vi "Main.vi"() -> ()   [LabVIEW 2021, in "Game of Life.lvlib"]
doc: "This template is for the Queued Message Handler design pattern.\n\nThe Event Handling Loop generates messages based on user interface actions.\n\nThe Message Handling Loop processes messages generated by the Event Handling Loop, or by other messages. The messages are string values, so new messages can be added easily to the Message Cases case structure in the Message Handling Loop. Each message cluster can also provide an optional value for Message Data, which is a variant that can be converted to whatever message-specific data is required."
uses:
  Game of Life.lvlib
  <vilib>/Plug-In SDKs/InstrumentStudio SDK/InstrumentStudioPluginSDK.lvlibp/Plugin Events Enum.ctl
  controls/Data.ctl
  controls/Configuration.ctl
  <vilib>/Utility/error.llb/DialogType.ctl
  controls/Game of Life.ctl
  a2cd5499-92a9-455c-b0f9-1db12e3f6067.vi
  aef85ed4-6d5b-4a62-8cd4-232f16e6ae51.vi
  a2cd5499-92a9-455c-b0f9-1db12e3f6067.vi/6651a77e-856e-4bcd-af5a-c0c13b264cc1.vi
  aef85ed4-6d5b-4a62-8cd4-232f16e6ae51.vi/331b549c-fcf8-43d9-8a1e-5b3c0091a99c.vi
  <vilib>/JDP Science/JSONtext/JSON text to Variant.vi
  <vilib>/Utility/error.llb/Error Cluster From Error Code.vi
  <vilib>/JDP Science/JSONtext/Variant to JSON Text.vi
  <vilib>/JDP Science/JSONtext/LVClass Serializer/JSONtext LVClass Serializer.lvclass
  <vilib>/ErrorRing/Error Ring.xnode
  <vilib>/Plug-In SDKs/InstrumentStudio SDK/InstrumentStudioPluginSDK.lvlibp/Plugin Session.lvclass
  <vilib>/Plug-In SDKs/InstrumentStudio SDK/InstrumentStudioPluginSDK.lvlibp
panel:
  in  "Tab Control":enum32{"Game Panel", "Events"}(tab)
  in  "Start/Stop":bool
  out "game of life":T1(graph)
  out "generation":u32 caption="Generation"
  in  "update interval":u32=250 caption="Update interval (msec)" min=50 max=1000
  in  "height":u32=100 caption="Board height" min=10
  in  "width":u32=100 caption="Board width" min=10
  in  "Log Events?":bool caption="Enable Logging"
  out "Event Record":i32(listbox)
  out "Log file directory":path
  in  "Session Id":u64
  # "When logging is enabled, a log file will be generated in the specified \ndirectory after the front panel is closed."
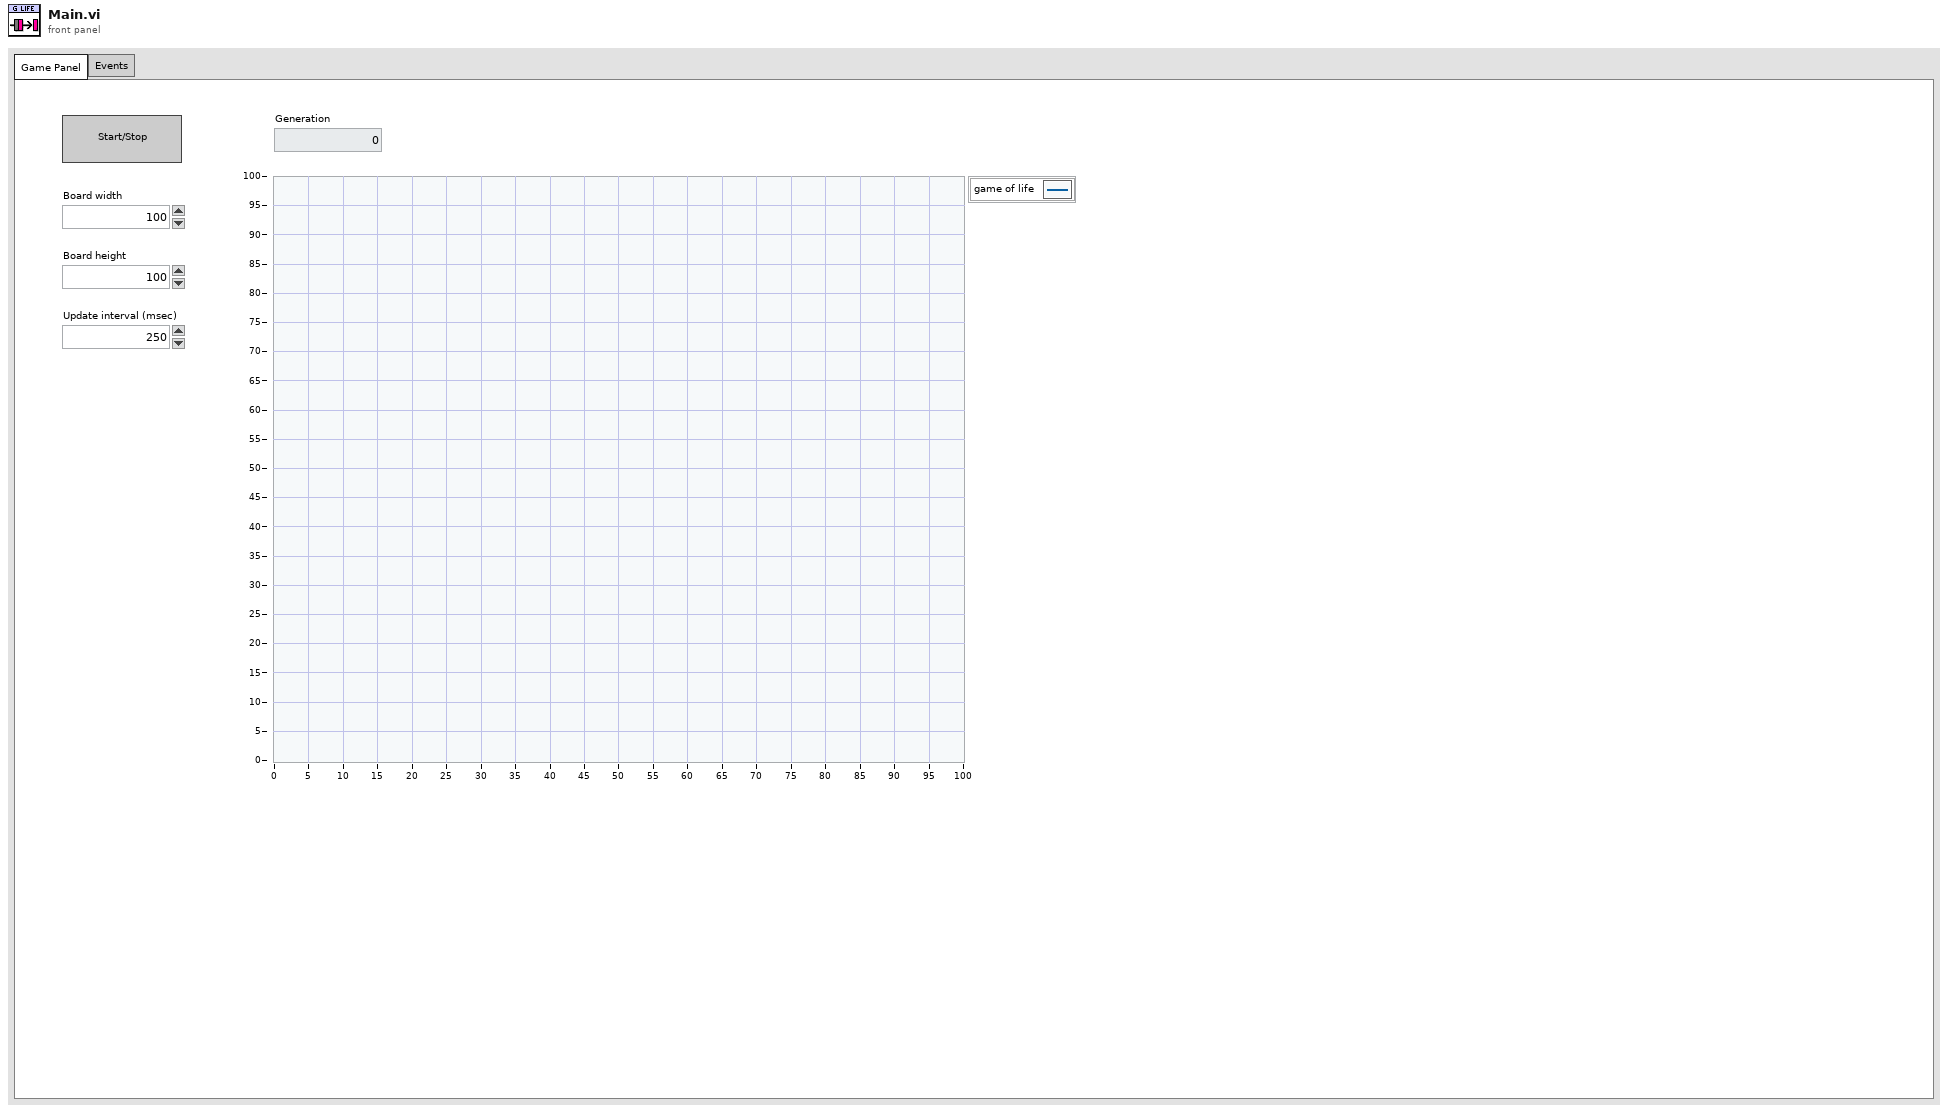
[diagram p1: front panel]
types:
  T1 = typedef "Game of Life.lvlib/Game of Life.ctl" = cluster{"x_data":dbl[], "y_data":dbl[]}
  T2 = typedef "Game of Life.lvlib/Data.ctl" = cluster{"Configuration":T3, "Generation":u32, "Item Names":string[], "Run?":bool, "Cells":bool[][]}
  T3 = typedef "Game of Life.lvlib/Configuration.ctl" = cluster{"Height":u32, "Width":u32, "Interval":u32, "Log Path":path, "Log Events?":bool}
  T4 = typedef "InstrumentStudioPluginSDK.lvlibp/Plugin Events Enum.ctl" = enum16{"Shutdown", "Project Saved", "Stop All Outputs"}
  T5 = typedef "InstrumentStudioPluginSDK.lvlibp/Event Registration Refnum.ctl" = refnum<event-registration>
  T6 = typedef "Game of Life.lvlib/All Message Queues.ctl" = cluster{"UI":refnum<queue>}
  T7 = cluster{"Event Refnum":T5, "Event Registration Refnum":refnum<event-registration>}
  T8 = enum8{"Enabled", "Disabled", "Disabled and Grayed Out"}
  T9 = typedef "DialogType.ctl" = u16
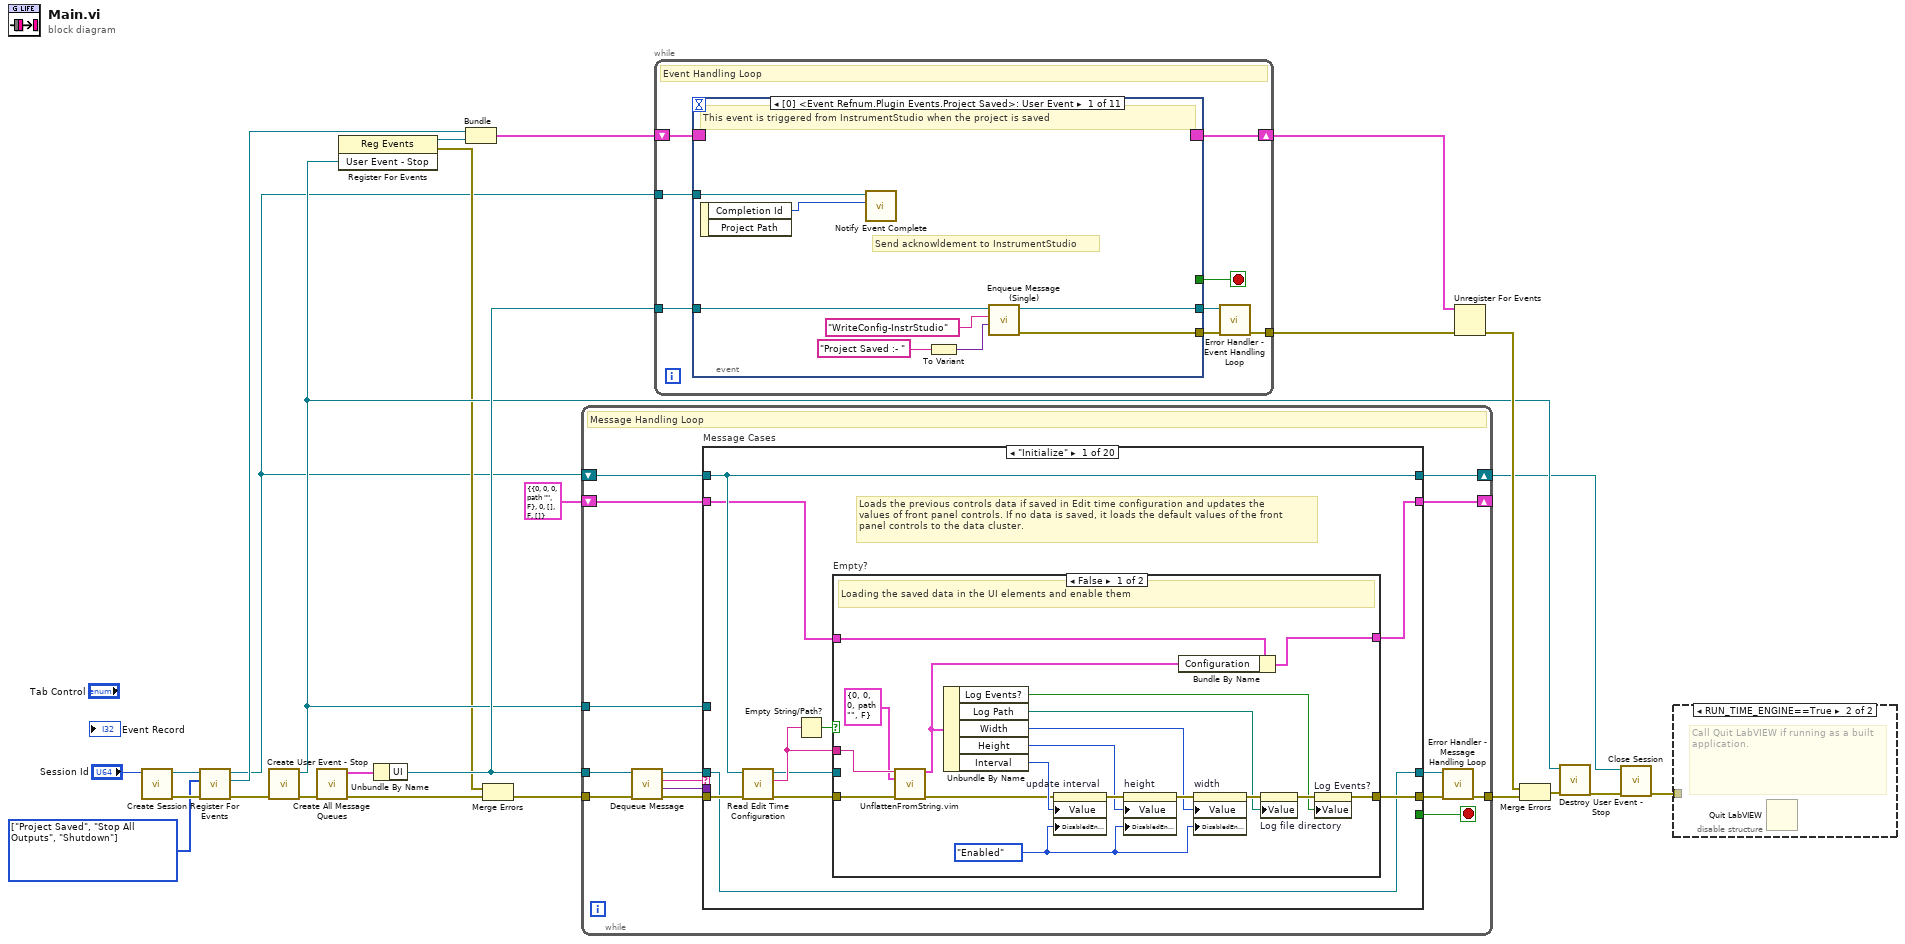
[diagram p0: block diagram]
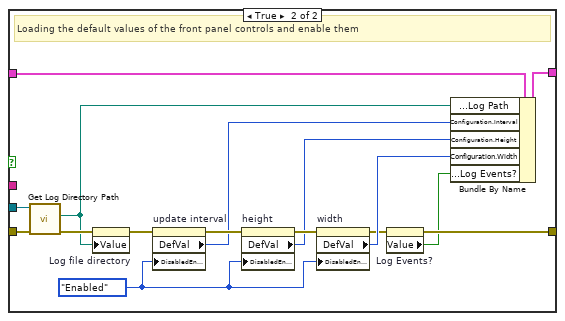
[diagram p3: hidden frame]
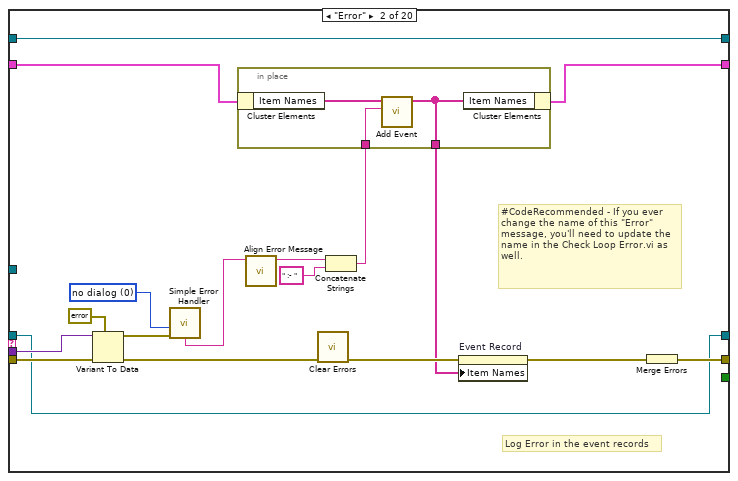
[diagram p4: hidden frame]
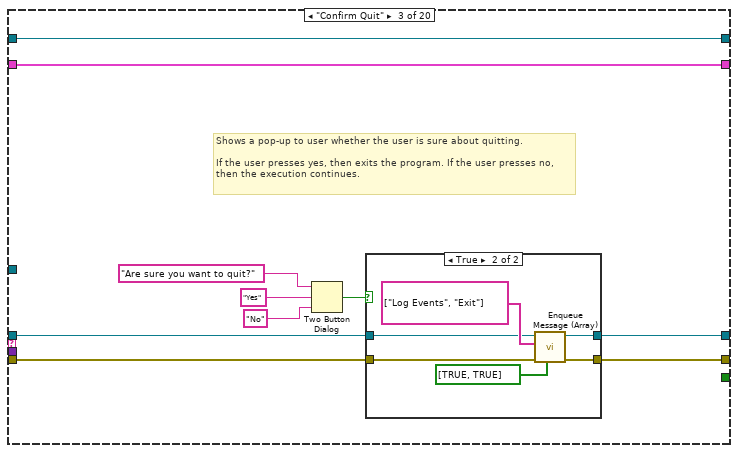
[diagram p5: hidden frame]
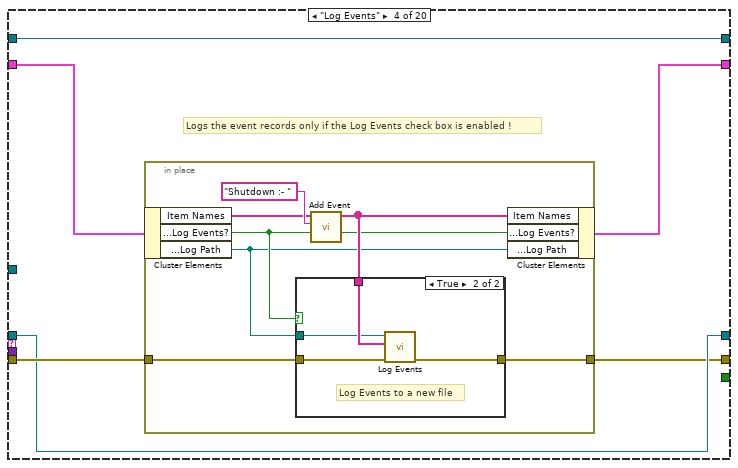
[diagram p7: hidden frame]
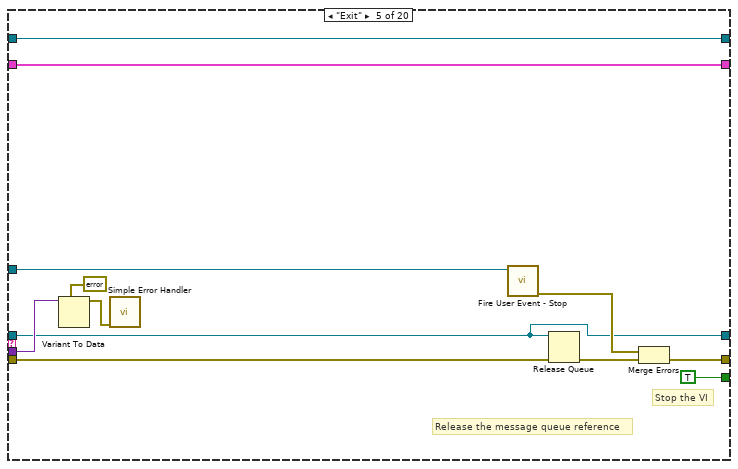
[diagram p9: hidden frame]
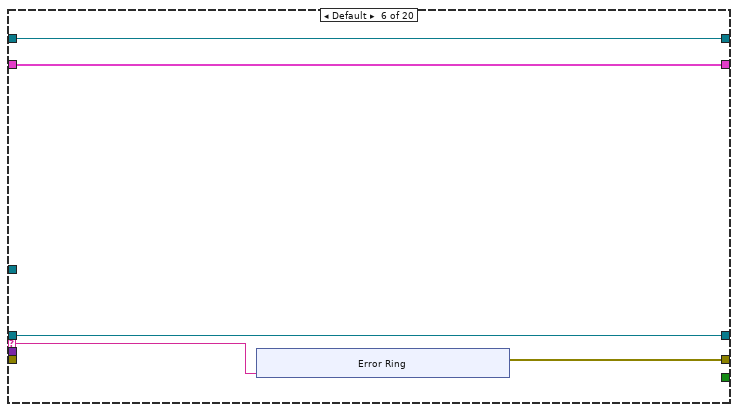
[diagram p10: hidden frame]
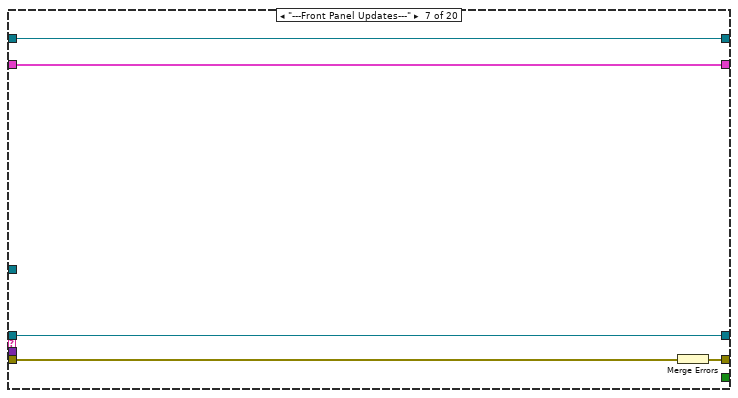
[diagram p11: hidden frame]
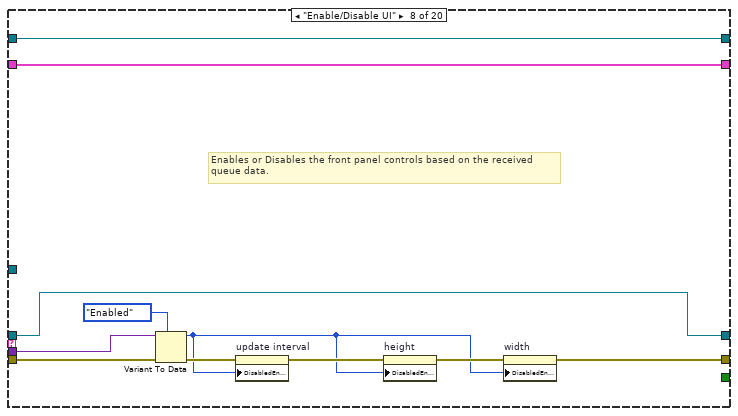
[diagram p12: hidden frame]
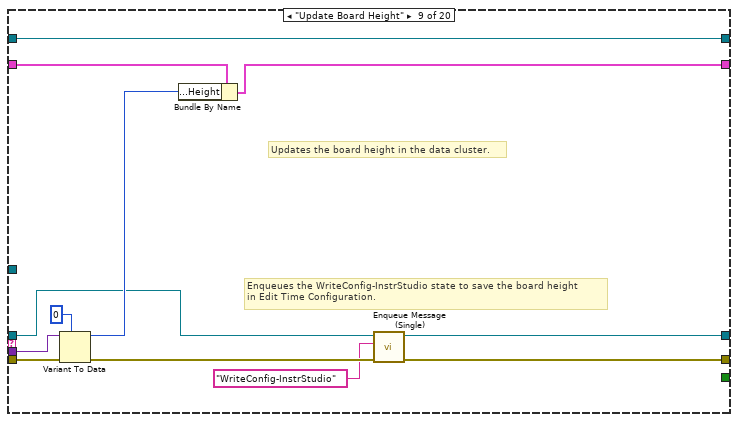
[diagram p13: hidden frame]
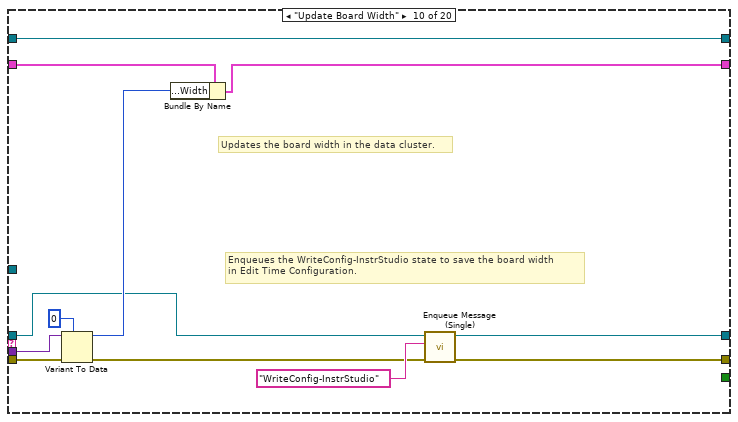
[diagram p14: hidden frame]
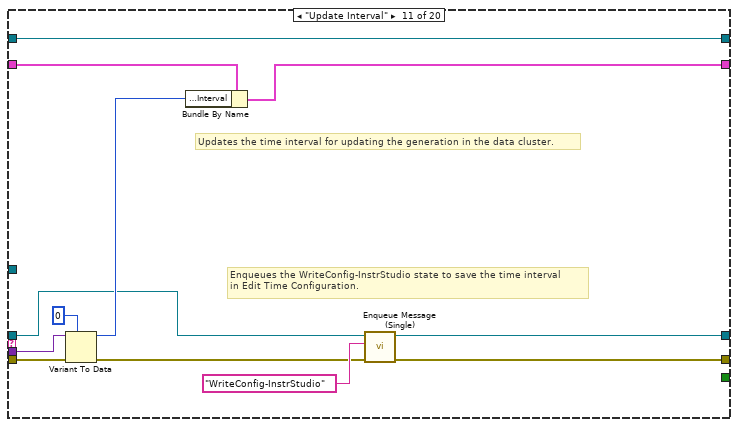
[diagram p15: hidden frame]
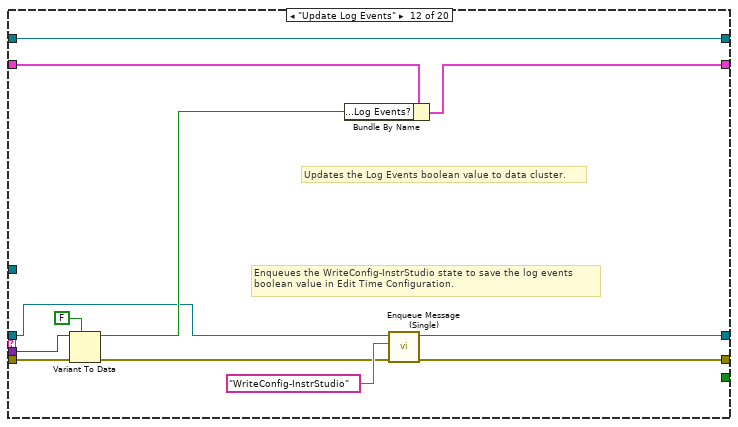
[diagram p16: hidden frame]
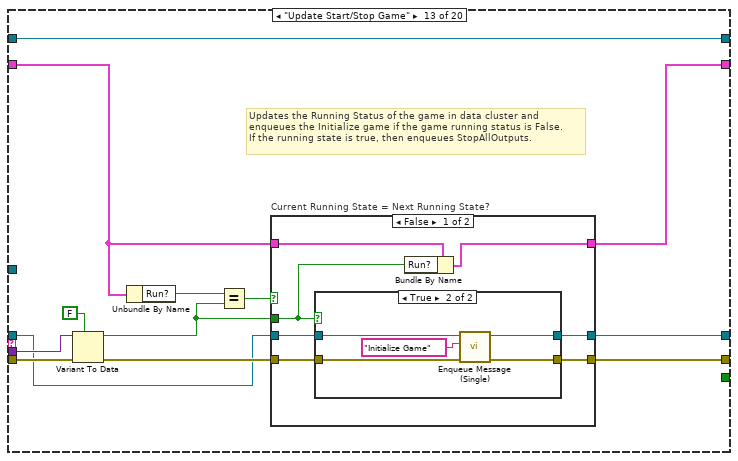
[diagram p17: hidden frame]
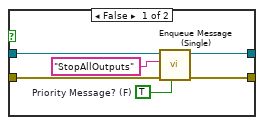
[diagram p18: hidden frame]
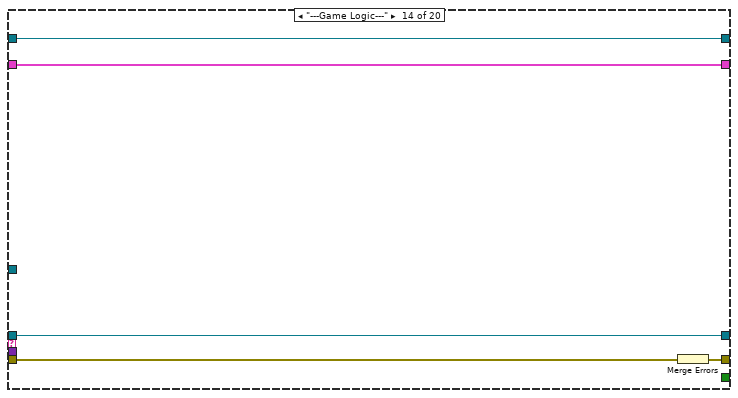
[diagram p20: hidden frame]
diagram:
  w9 = T4[] [enum."Project Saved", enum."Stop All Outputs", enum."Shutdown"] items=["Shutdown", "Project Saved", "Stop All Outputs"] ("Events To Register")
  n1 = call <vilib>:"Create Session.vi"("Session Id"="Session Id") -> ("error out"=w12:errorcluster, "Session out"=w10:refnum<class "Plugin Session.lvclass">)  [unwired: 6 in, 3 out]
  n2 = call <vilib>:"Register For Events.vi"("error in (no error)"=w12, "Events To Register"=w9, "Session in"=w10) -> ("error out"=w11:errorcluster, "Event Refnum"=w6:T5, "Session out"=w2:refnum<class "Plugin Session.lvclass">)  [unwired: 6 in]
  n3 = call "Create User Event - Stop.vi"("error in (no error)"=w11) -> ("error out"=w21:errorcluster, "User Event - Stop"=w16:refnum<user-event>)  [unwired: 9 in]
  n4 = call "Create All Message Queues.vi"("error in (no error)"=w21) -> ("error out"=w25:errorcluster, "Message Queues out"=w24:T6)  [unwired: 9 in]
  n5 = register-events(w16) -> (reference out=w8:refnum<event-registration>, error out=w14:errorcluster)  [unwired: 2 in]
  n6 = Unbundle By Name(w24) -> ("UI"=w22:refnum<queue>)
  n7 = Bundle("Event Refnum"=w6, "Event Registration Refnum"=w8) -> (w7:T7)  [unwired: 1 in]
  n8 = Merge Errors(w14, w25) -> (w15:errorcluster)
  n9 = while {
    tunnel: w22 -> [w34]
    tunnel: w16 -> [w39]
    tunnel: w15 -> [w38]
    tunnel: [w32] -> w23
    shift-right: [w29] -> w5
    shift-left: w2 -> [w30]
    shift-right: [w28] -> _
    shift-left: T2 {"Configuration"={"Height"=0, "Width"=0, "Interval"=0, "Log Path"=path "", "Log Events?"=FALSE}, "Generation"=0, "Item Names"=[], "Run?"=FALSE, "Cells"=[]} ("Configuration") -> [w27]
    stop <- w40 stop-if-true
    # "Message Handling Loop"
    n10 = call "Dequeue Message.vi"("error in (no error)"=w38, "Message Queue"=w34) -> ("error out"=w37:errorcluster, "Message Data"=w35:variant, "Message"=w36:string, "dup Message Queue"=w33:refnum<queue>)  [unwired: 6 in]
    n11 = case "Message Cases" shown="\"Initialize\"" w36 {
      selector: w36 -> [_ _ _ _ _ w157 _ _ _ _ _ _ _ _ _ _ _ _ _ _]
      tunnel: w33 -> [w44 w95 w113 w128 w143 w154 w166 w171 w183 w195 w206 w219 w230 w264 w283 w294 w329 w348 w355 w372]
      tunnel: w37 -> [w46 w102 w115 w129 w142 _ w170 w175 w192 w204 w216 w228 w236 w268 w281 w298 w333 w335 w356 w371]
      tunnel: [w50 w97 w114 w124 w151 w158 w169 w177 w185 w194 w208 w220 w239 w267 w269 w295 w332 w346 w357 w376] -> w31
      tunnel: [_ _ _ _ TRUE _ _ _ _ _ _ _ _ _ _ _ _ _ _ _] -> w40
      tunnel: w35 -> [_ w101 _ _ w146 _ _ w174 w191 w203 w215 w227 w235 _ _ _ _ _ _ w361]
      tunnel: w39 -> [_ _ _ _ w150 _ _ _ _ _ _ _ _ _ _ _ _ _ _ _]
      tunnel: w30 -> [w45 w96 w112 w127 w145 w156 w168 w181 w193 w205 w217 w229 w242 w266 w287 w299 w331 w352 w359 w367]
      tunnel: [w45 w96 w112 w127 w145 w156 w168 w181 w193 w205 w217 w229 w242 w266 w287 w299 w331 w352 w358 w377] -> w29
      tunnel: [w43 w92 w111 w126 w144 w155 w167 w180 w188 w201 w213 w225 w240 w265 w286 w288 w330 w350 w354 w366] -> w28
      tunnel: w27 -> [w42 w91 w111 w125 w144 w155 w167 w180 w187 w200 w212 w224 w241 w265 w285 w292 w330 w339 w354 w365]
      tunnel: [w44 w95 w110 w128 w143 w154 w166 w171 w184 w196 w207 w218 w238 w264 w282 w291 w329 w344 w355 w372] -> w26
      frame "Initialize" {
        # "Loads the previous controls data if saved in Edit time configuration and updates the\nvalues of front panel controls. If no data is saved, it loads the default values of the front\npanel controls to the data cluster."
        # "Initialize - All initialization work should take place in this message, since other loops can potentially enqueue messages that execute immediately after this one."
        n12 = call <vilib>:"Read Edit Time Configuration.vi"("error in (no error)"=w46, "Session in"=w45) -> ("error out"=w47:errorcluster, "Edit Time Configuration"=w48:string, "Session out"=w41:refnum<class "Plugin Session.lvclass">)  [unwired: 7 in]
        n13 = Empty String/Path?(string/path=w48) -> (empty?=w49:bool)
        n14 = case "Empty?" shown="False" w49 {
          tunnel: [w52 w70] -> w50
          tunnel: w47 -> [w67 w74]
          tunnel: w48 -> [w68 _]
          tunnel: w42 -> [w60 w84]
          tunnel: [w59 w80] -> w43
          tunnel: w41 -> [_ w72]
          frame False {
            w56 = T8."Enabled" ("Disabled")
            # "Loading the saved data in the UI elements and enable them"
            n15 = call "UnflattenFromString.vim"("Flattened Data"=w68, "Data Type"=T3 {"Height"=0, "Width"=0, "Interval"=0, "Log Path"=path "", "Log Events?"=FALSE} ("Configuration"), "error in"=w67) -> ("Data Out"=w58:T3, "error out"=w57:errorcluster)  [unwired: 11 in]
            n16 = Unbundle By Name(w58) -> ("Log Events?"=w51:bool, "Log Path"=w54:path, "Width"=w62:u32, "Height"=w64:u32, "Interval"=w66:u32)
            n17 = property on="update interval" class="DigNum (strict)"(error in=w57, "Value"=w66, "DisabledEnum"=w56) -> (error out=w65:errorcluster)  [unwired: 1 in, 1 out]
            n18 = property on="height" class="DigNum (strict)"(error in=w65, "Value"=w64, "DisabledEnum"=w56) -> (error out=w63:errorcluster)  [unwired: 1 in, 1 out]
            n19 = Bundle By Name(cluster=w60, "Configuration"=w58) -> (w59:T2)
            n20 = property on="width" class="DigNum (strict)"(error in=w63, "Value"=w62, "DisabledEnum"=w56) -> (error out=w55:errorcluster)  [unwired: 1 in, 1 out]
            n21 = property on="Log file directory" class="Path"(error in=w55, "Value"=w54) -> (error out=w53:errorcluster)  [unwired: 1 in, 1 out]
            n22 = property on="Log Events?" class="Bool (strict)"(error in=w53, "Value"=w51) -> (error out=w52:errorcluster)  [unwired: 1 in, 1 out]
          }
          frame True {
            w77 = T8."Enabled" ("Disabled")
            # "Loading the default values of the front panel controls and enable them"
            n23 = call "Get Log Directory Path.vi"("error in (no error)"=w74, "Plugin Session in"=w72) -> ("error out"=w75:errorcluster, "Log file directory path"=w73:path)  [unwired: 7 in, 1 out]
            n24 = property on="Log file directory" class="Path"(error in=w75, "Value"=w73) -> (error out=w76:errorcluster)  [unwired: 1 in, 1 out]
            n25 = property on="update interval" class="DigNum (strict)"(error in=w76, "DisabledEnum"=w77) -> (error out=w83:errorcluster, "DefVal"=w81:u32)  [unwired: 1 in, 1 out]
            n26 = property on="height" class="DigNum (strict)"(error in=w83, "DisabledEnum"=w77) -> (error out=w82:errorcluster, "DefVal"=w79:u32)  [unwired: 1 in, 1 out]
            n27 = property on="width" class="DigNum (strict)"(error in=w82, "DisabledEnum"=w77) -> (error out=w71:errorcluster, "DefVal"=w78:u32)  [unwired: 1 in, 1 out]
            n28 = property on="Log Events?" class="Bool (strict)"(error in=w71) -> (error out=w70:errorcluster, "Value"=w69:bool)  [unwired: 1 in, 1 out]
            n29 = Bundle By Name(cluster=w84, "Configuration.Log Path"=w73, "Configuration.Interval"=w81, "Configuration.Height"=w79, "Configuration.Width"=w78, "Configuration.Log Events?"=w69) -> (w80:T2)
          }
        }
      }
      frame "Error" {
        w94 = T9 0 items=["no dialog", "OK message", "continue or stop message", "OK message + warnings", "continue/stop + warnings"] ("type of dialog (OK msg:1)")
        # "#CodeRecommended - If you ever change the name of this \"Error\" message, you'll need to update the name in the Check Loop Error.vi as well."
        # "Log Error in the event records"
        # "Error - Display an error dialog. This message is sent by the \"Error Handler\" VIs at the end of other loops in this application."
        n30 = Variant To Data(error in=w102, type=errorcluster {"status"=FALSE, "code"=0, "source"=""} ("error constant"), Variant=w101) -> (data=w99:errorcluster, error out=w98:errorcluster)
        n31 = call <vilib>:"Simple Error Handler.vi"("type of dialog (OK msg:1)"=w94, "error in (no error)"=w99) -> ("message"=w86:string)  [unwired: 3 in, 4 out]
        n32 = call "Align Error Message.vi"("Message in"=w86) -> ("Message out"=w85:string)  [unwired: 10 in]
        n33 = call <vilib>:"Clear Errors.vi"("error in (no error)"=w98) -> ("error out"=w90:errorcluster)  [unwired: 5 in, 1 out]
        n34 = Concatenate Strings(w85, " :- " ("string")) -> (w93:string)
        n35 = in-place {
          in-place-border: w93 -> [w105]
          in-place-border: [w103] -> w88
          n36 = in-place-cluster #1(w91) -> ("Item Names"=w104:string[])
          n37 = call "Add Event.vi"("Event Tag"=w105, "Item Names in"=w104) -> ("Item Names out"=w103:string[])  [unwired: 9 in]
          n38 = in-place-cluster #1("Item Names"=w103) -> (w92:T2)
        }
        n39 = property on="Event Record" class="LstBox (strict)"(error in=w90, "Item Names"=w88) -> (error out=w89:errorcluster)  [unwired: 1 in, 1 out]
        n40 = Merge Errors(w89) -> (w97:errorcluster)
      }
      frame "Confirm Quit" {
        # "Shows a pop-up to user whether the user is sure about quitting. \n\nIf the user presses yes, then exits the program. If the user presses no,\nthen the execution continues."
        # "Confirm Quit - Message that can confirm whether or not the user wants to exit the application."
        n41 = Two Button Dialog(message="Are sure you want to quit?", 1:"No" ("F button name (\"Cancel\")"), 2:"Yes" ("T button name (\"OK\")")) -> (T button?=w106:bool)
        n42 = case shown="True" w106 {
          tunnel: w115 -> [w116 w119]
          tunnel: [w116 w120] -> w114
          tunnel: w113 -> [w117 w121]
          tunnel: [w117 w118] -> w110
          frame False {
          }
          frame True {
            n43 = call "Enqueue Message (Array).vi"("Priority Message? Array"=bool[] [TRUE, TRUE], "error in (no error)"=w119, "Message Array"=string[] ["Log Events", "Exit"], "Message Queue"=w121) -> ("error out"=w120:errorcluster, "dup Message Queue"=w118:refnum<queue>)  [unwired: 6 in]
          }
        }
      }
      frame "Log Events" {
        # "Logs the event records only if the Log Events check box is enabled !"
        n44 = in-place {
          in-place-border: w129 -> [w135]
          in-place-border: [w134] -> w124
          n45 = in-place-cluster #2(w125) -> ("Item Names"=w133:string[], "Configuration.Log Events?"=w131:bool, "Configuration.Log Path"=w130:path)
          n46 = call "Add Event.vi"("Event Tag"="Shutdown :- ", "Item Names in"=w133) -> ("Item Names out"=w132:string[])  [unwired: 9 in]
          n47 = case shown="True" w131 {
            tunnel: w135 -> [w137 w141]
            tunnel: [w137 w140] -> w134
            tunnel: w132 -> [_ w139]
            tunnel: w130 -> [_ w138]
            frame False {
            }
            frame True {
              # "Log Events to a new file"
              n48 = call "Log Events.vi"("error in"=w141, "Item Names"=w139, "Event Folder Path"=w138) -> ("error out"=w140:errorcluster)  [unwired: 8 in]
            }
          }
          n49 = in-place-cluster #2("Item Names"=w132, "Configuration.Log Events?"=w131, "Configuration.Log Path"=w130) -> (w126:T2)
        }
      }
      frame "Exit" {
        # "Stop the VI"
        # "Release the message queue reference"
        # "Exit - Exit the application."
        n50 = Variant To Data(type=errorcluster {"status"=FALSE, "code"=0, "source"=""} ("error constant"), Variant=w146) -> (data=w147:errorcluster)  [unwired: 1 in, 1 out]
        n51 = call <vilib>:"Simple Error Handler.vi"("error in (no error)"=w147) -> ()  [unwired: 4 in, 5 out]
        n52 = call "Fire User Event - Stop.vi"("User Event - Stop"=w150) -> ("error out"=w149:errorcluster)  [unwired: 10 in]
        n53 = Release Queue(queue=w143, error in (no error)=w142) -> (error out=w152:errorcluster)  [unwired: 1 in, 2 out]
        n54 = Merge Errors(w149, w152) -> (w151:errorcluster)
      }
      frame Default {
        # "'Default' case only runs if there is a message that isn't defined in any of the other cases.  Output a programming error."
        n55 = xnode "Error Ring"("parameter 0"=w157) -> ("error out"=w158:errorcluster)
      }
      frame "---Front Panel Updates---" {
        # "Duplicate this frame when creating new messages.  Change this comment in the duplicated frame to describe this message."
        n56 = Merge Errors(w170) -> (w169:errorcluster)
      }
      frame "Enable/Disable UI" {
        # "Enables or Disables the front panel controls based on the received \nqueue data."
        n57 = Variant To Data(error in=w175, type=T8."Enabled" ("Disabled"), Variant=w174) -> (data=w172:T8, error out=w176:errorcluster)
        n58 = property on="update interval" class="DigNum (strict)"(error in=w176, "DisabledEnum"=w172) -> (error out=w179:errorcluster)  [unwired: 1 in, 1 out]
        n59 = property on="height" class="DigNum (strict)"(error in=w179, "DisabledEnum"=w172) -> (error out=w178:errorcluster)  [unwired: 1 in, 1 out]
        n60 = property on="width" class="DigNum (strict)"(error in=w178, "DisabledEnum"=w172) -> (error out=w177:errorcluster)  [unwired: 1 in, 1 out]
      }
      frame "Update Board Height" {
        # "Enqueues the WriteConfig-InstrStudio state to save the board height\nin Edit Time Configuration."
        # "Updates the board height in the data cluster."
        n61 = Variant To Data(error in=w192, type=u32 0 ("wid"), Variant=w191) -> (data=w189:u32, error out=w186:errorcluster)
        n62 = Bundle By Name(cluster=w187, "Configuration.Height"=w189) -> (w188:T2)
        n63 = call "Enqueue Message (Single).vi"("error in (no error)"=w186, "Message"="WriteConfig-InstrStudio", "Message Queue"=w183) -> ("error out"=w185:errorcluster, "dup Message Queue"=w184:refnum<queue>)  [unwired: 7 in]
      }
      frame "Update Board Width" {
        # "Enqueues the WriteConfig-InstrStudio state to save the board width\nin Edit Time Configuration."
        # "Updates the board width in the data cluster."
        n64 = Variant To Data(error in=w204, type=u32 0 ("wid"), Variant=w203) -> (data=w199:u32, error out=w197:errorcluster)
        n65 = Bundle By Name(cluster=w200, "Configuration.Width"=w199) -> (w201:T2)
        n66 = call "Enqueue Message (Single).vi"("error in (no error)"=w197, "Message"="WriteConfig-InstrStudio", "Message Queue"=w195) -> ("error out"=w194:errorcluster, "dup Message Queue"=w196:refnum<queue>)  [unwired: 7 in]
      }
      frame "Update Interval" {
        # "Enqueues the WriteConfig-InstrStudio state to save the time interval\nin Edit Time Configuration."
        # "Updates the time interval for updating the generation in the data cluster."
        n67 = Variant To Data(error in=w216, type=u32 0 ("wid"), Variant=w215) -> (data=w211:u32, error out=w209:errorcluster)
        n68 = Bundle By Name(cluster=w212, "Configuration.Interval"=w211) -> (w213:T2)
        n69 = call "Enqueue Message (Single).vi"("error in (no error)"=w209, "Message"="WriteConfig-InstrStudio", "Message Queue"=w206) -> ("error out"=w208:errorcluster, "dup Message Queue"=w207:refnum<queue>)  [unwired: 7 in]
      }
      frame "Update Log Events" {
        # "Enqueues the WriteConfig-InstrStudio state to save the log events\nboolean value in Edit Time Configuration."
        # "Updates the Log Events boolean value to data cluster."
        n70 = Variant To Data(error in=w228, type=FALSE, Variant=w227) -> (data=w223:bool, error out=w221:errorcluster)
        n71 = Bundle By Name(cluster=w224, "Configuration.Log Events?"=w223) -> (w225:T2)
        n72 = call "Enqueue Message (Single).vi"("error in (no error)"=w221, "Message"="WriteConfig-InstrStudio", "Message Queue"=w219) -> ("error out"=w220:errorcluster, "dup Message Queue"=w218:refnum<queue>)  [unwired: 7 in]
      }
      frame "Update Start/Stop Game" {
        # "Updates the Running Status of the game in data cluster and\nenqueues the Initialize game if the game running status is False.\nIf the running state is true, then enqueues StopAllOutputs."
        n73 = Variant To Data(error in=w236, type=FALSE, Variant=w235) -> (data=w233:bool, error out=w237:errorcluster)
        n74 = Unbundle By Name(w241) -> ("Run?"=w232:bool)
        n75 = Equal?(x=w232, y=w233) -> (x = y?=w231:bool)
        n76 = case "Current Running State = Next Running State?" shown="False" w231 {
          tunnel: w237 -> [w245 w262]
          tunnel: w241 -> [w249 w263]
          tunnel: [w248 w263] -> w240
          tunnel: [w246 w262] -> w239
          tunnel: w230 -> [w247 w261]
          tunnel: [w244 w261] -> w238
          tunnel: w233 -> [w243 _]
          frame False {
            n77 = case shown="True" w243 {
              tunnel: w247 -> [w253 w260]
              tunnel: [w251 w259] -> w246
              tunnel: w245 -> [w252 w258]
              tunnel: [w250 w257] -> w244
              frame False {
                w255 = TRUE  # Priority Message? (F)
                n78 = call "Enqueue Message (Single).vi"("Priority Message? (F)"=w255, "error in (no error)"=w252, "Message"="StopAllOutputs", "Message Queue"=w253) -> ("error out"=w251:errorcluster, "dup Message Queue"=w250:refnum<queue>)  [unwired: 6 in]
              }
              frame True {
                n79 = call "Enqueue Message (Single).vi"("error in (no error)"=w258, "Message"="Initialize Game", "Message Queue"=w260) -> ("error out"=w259:errorcluster, "dup Message Queue"=w257:refnum<queue>)  [unwired: 7 in]
              }
            }
            n80 = Bundle By Name(cluster=w249, "Run?"=w243) -> (w248:T2)
          }
          frame True {
          }
        }
      }
      frame "---Game Logic---" {
        # "Duplicate this frame when creating new messages.  Change this comment in the duplicated frame to describe this message."
        n81 = Merge Errors(w268) -> (w267:errorcluster)
      }
      frame "Initialize Game" {
        w280 = -1.0 ("X Scale.Range:Minimum")
        # "Generate an initial random \nliving cells in a 2D array"
        # "Initializes the Board"
        n82 = Unbundle By Name(w285) -> ("Configuration.Width"=w278:u32, "Configuration.Height"=w276:u32)
        n83 = To Double Precision Float(number=w278) -> (double precision float=w279:dbl)
        n84 = To Double Precision Float(number=w276) -> (double precision float=w277:dbl)
        n85 = call "Initialize Game.vi"("Height"=w276, "Width"=w278) -> ("Array"=w284:bool[][])  [unwired: 9 in]
        n86 = property on="game of life" class="XYGraph (strict)"(error in=w281, "XScale.Minimum"=w280, "XScale.Maximum"=w279, "YScale.Minimum"=w280, "YScale.Maximum"=w277, "Value"=T1 {"x_data"=[], "y_data"=[]} ("game of life")) -> (error out=w275:errorcluster)  [unwired: 1 in, 1 out]
        n87 = Bundle By Name(cluster=w285, "Generation"=u32 0, "Cells"=w284) -> (w286:T2)
        n88 = call "Enum to Variant Array.vi"("Disabled"=T8."Disabled and Grayed Out") -> ("Message Data Array"=w270:variant[])  [unwired: 10 in]
        n89 = call "Enqueue Message (Array).vi"("error in (no error)"=w275, "Message Data Array"=w270, "Message Array"=string[] ["Enable/Disable UI", "UpdateRunningFlag-InstrStudio", "Game of Life"], "Message Queue"=w283) -> ("error out"=w269:errorcluster, "dup Message Queue"=w282:refnum<queue>)  [unwired: 6 in]
      }
      frame "Game of Life" {
        # "If the stop condition is met, then stops execution of the \ngame logic. If not, keeps executing the game logic by \nenqueueing the present state."
        # "Generates the next generation of living cells by\nappliying game logic to the current generation \nliving cells with the specified time interval."
        n90 = in-place {
          in-place-border: w298 -> [w308]
          in-place-border: [w304] -> w296
          in-place-border: [w303] -> w297
          in-place-border: [w302] -> w293
          in-place-border: [w300] -> w290
          n91 = in-place-cluster #3(w292) -> ("Cells"=w307:bool[][], "Generation"=w306:u32, "Configuration.Interval"=w301:u32)
          n92 = call "Wrap Next Generation.vi"("error in"=w308, "Update Interval"=w301, "generation in"=w306, "cells in"=w307) -> ("error out"=w304:errorcluster, "game of life"=w302:T1, "generation out"=w300:u32, "cells out"=w305:bool[][], "Stop?"=w303:bool)  [unwired: 3 in]
          n93 = in-place-cluster #3("Cells"=w305, "Generation"=w300, "Configuration.Interval"=w301) -> (w289:T2)
        }
        n94 = case "Stop?" shown="True" w297 {
          tunnel: w296 -> [w313 w319]
          tunnel: [w316 w325] -> w295
          tunnel: w294 -> [w315 w324]
          tunnel: w293 -> [w310 _]
          tunnel: [w312 w323] -> w291
          tunnel: w290 -> [w311 _]
          tunnel: w289 -> [w309 w321]
          tunnel: [w309 w322] -> w288
          frame False {
            n95 = call "Enqueue Message (Single).vi"("error in (no error)"=w313, "Message"="Game of Life", "Message Queue"=w315) -> ("error out"=w316:errorcluster, "dup Message Queue"=w312:refnum<queue>)  [unwired: 7 in]
            "generation" <- w311
            "game of life" <- w310
          }
          frame True {
            n96 = property on="Start/Stop" class="Bool (strict)"(error in=w319, "Value"=FALSE ("Start/Stop")) -> (error out=w318:errorcluster)  [unwired: 1 in, 1 out]
            n97 = call "Enum to Variant Array.vi"("Disabled"=T8."Enabled") -> ("Message Data Array"=w328:variant[])  [unwired: 10 in]
            n98 = Bundle By Name(cluster=w321, "Run?"=FALSE) -> (w322:T2)
            n99 = call "Enqueue Message (Array).vi"("error in (no error)"=w318, "Message Data Array"=w328, "Message Array"=string[] ["Enable/Disable UI", "UpdateRunningFlag-InstrStudio"], "Message Queue"=w324) -> ("error out"=w325:errorcluster, "dup Message Queue"=w323:refnum<queue>)  [unwired: 6 in]
          }
        }
      }
      frame "---Instrument Studio Interaction---" {
        # "Duplicate this frame when creating new messages.  Change this comment in the duplicated frame to describe this message."
        n100 = Merge Errors(w333) -> (w332:errorcluster)
      }
      frame "StopAllOutputs" {
        # "Flush the Queue to stop game logic execution"
        # "Updates the Running Status of the game in data cluster"
        # "Updates the Event Record indicator with current event."
        n101 = Unbundle By Name(w339) -> ("Item Names"=w338:string[])
        n102 = property on="Start/Stop" class="Bool (strict)"(error in=w335, "Value"=FALSE ("Start/Stop")) -> (error out=w336:errorcluster)  [unwired: 1 in, 1 out]
        n103 = call "Add Event.vi"("Event Tag"="Stop All Outputs :- ", "Item Names in"=w338) -> ("Item Names out"=w337:string[])  [unwired: 9 in]
        n104 = property on="Event Record" class="LstBox (strict)"(error in=w336, "Item Names"=w337) -> (error out=w349:errorcluster)  [unwired: 1 in, 1 out]
        n105 = Bundle By Name(cluster=w339, "Item Names"=w337, "Run?"=FALSE) -> (w350:T2)
        n106 = Flush Queue(queue=w348, error in (no error)=w349) -> (queue out=w345:refnum<queue>, error out=w347:errorcluster)  [unwired: 1 out]
        n107 = call "Enum to Variant Array.vi"("Disabled"=T8."Enabled") -> ("Message Data Array"=w341:variant[])  [unwired: 10 in]
        n108 = call "Enqueue Message (Array).vi"("error in (no error)"=w347, "Message Data Array"=w341, "Message Array"=string[] ["Enable/Disable UI", "UpdateRunningFlag-InstrStudio"], "Message Queue"=w345) -> ("error out"=w346:errorcluster, "dup Message Queue"=w344:refnum<queue>)  [unwired: 6 in]
      }
      frame "UpdateRunningFlag-InstrStudio" {
        # "Updates the running flag in \nInstrumentStudio"
        n109 = Unbundle By Name(w354) -> ("Run?"=w353:bool)
        n110 = call <vilib>:"Update Running State.vi"("error in (no error)"=w356, "Is Running"=w353, "Plugin Session in"=w359) -> ("error out"=w357:errorcluster, "Plugin Session out"=w358:refnum<class "Plugin Session.lvclass">)  [unwired: 7 in]
      }
      frame "WriteConfig-InstrStudio" {
        w362 = variant  # Empty Variant
        # "Saving the control inputs\nin the instrumentStudio object"
        n111 = Unbundle By Name(w365) -> ("Configuration"=w369:T3, "Item Names"=w364:string[])
        n112 = Equal?(x=w362, y=w361) -> (x = y?=w370:bool)
        n113 = case "Empty Variant?" shown="False" w370 {
          tunnel: [w382 w394] -> w373
          tunnel: [w391 w395] -> w363
          tunnel: w371 -> [w387 w394]
          tunnel: w361 -> [w386 _]
          tunnel: w364 -> [w390 w395]
          tunnel: w369 -> [w384 w392]
          tunnel: w367 -> [w381 w393]
          tunnel: [w380 w393] -> w368
          tunnel: [w379 w392] -> w360
          frame False {
            # "Gets the Log file\ndirectory path."
            # "Records the project save event in event record indicator."
            n114 = Variant To Data(error in=w387, type="", Variant=w386) -> (data=w385:string, error out=w388:errorcluster)
            n115 = call "Add Event.vi"("Event Tag"=w385, "Item Names in"=w390) -> ("Item Names out"=w391:string[])  [unwired: 9 in]
            n116 = property on="Event Record" class="LstBox (strict)"(error in=w388, "Item Names"=w391) -> (error out=w383:errorcluster)  [unwired: 1 in, 1 out]
            n117 = call "Get Log Directory Path.vi"("error in (no error)"=w383, "Plugin Session in"=w381) -> ("error out"=w382:errorcluster, "Log file directory path"=w378:path, "Plugin Session out"=w380:refnum<class "Plugin Session.lvclass">)  [unwired: 7 in]
            "Log file directory" <- w378
            n118 = Bundle By Name(cluster=w384, "Log Path"=w378) -> (w379:T3)
          }
          frame True {
          }
        }
        n119 = call "FlattenToString.vim"("Anything"=w360, "error in"=w373) -> ("Flattened Data"=w375:string, "error out"=w374:errorcluster)  [unwired: 12 in]
        n120 = Bundle By Name(cluster=w365, "Item Names"=w363, "Configuration"=w360) -> (w366:T2)
        n121 = call <vilib>:"Write Edit Time Configuration.vi"("error in (no error)"=w374, "Edit Time Configuration"=w375, "Session in"=w368) -> ("error out"=w376:errorcluster, "Session out"=w377:refnum<class "Plugin Session.lvclass">)  [unwired: 7 in]
      }
    }
    n122 = call "Error Handler - Message Handling Loop.vi"("error in (no error)"=w31, "Message Queue"=w26) -> ("dup error in"=w32:errorcluster)  [unwired: 8 in, 1 out]
  }
  n123 = while {
    tunnel: w22 -> [w403]
    shift-right: [w401] -> w18
    shift-left: w7 -> [w402]
    tunnel: [w397] -> w17
    tunnel: w2 -> [w396]
    stop <- w399 stop-if-true
    # "Event Handling Loop"
    n124 = event shown="[0] <Event Refnum.Plugin Events.Project Saved>: User Event" {
      selector: w402 -> [_ _ _ _ _ _ _ _ _ _ _]
      dyn-events: [_ _ _ _ _ _ _ _ _ _ _] -> w401
      timeout: _ -> [_ _ _ _ _ _ _ _ _ _ _]
      tunnel: [_ _ _ _ _ _ _ _ _ _ w464] -> w399
      tunnel: w403 -> [w408 w416 w421 w427 w433 w439 w444 w450 w457 w460 w465]
      tunnel: [w406 w413 w422 w426 w432 w438 _ w449 w456 w459 _] -> w400
      tunnel: [w407 w414 w423 w428 w434 w440 w443 w451 w455 w461 w465] -> w398
      tunnel: w396 -> [w411 w418 _ _ _ _ _ _ _ _ _]
      event User Event {
        # "Send acknowldement to InstrumentStudio"
        # "This event is triggered from InstrumentStudio when the project is saved"
        n125 = event-data() -> ("Completion Id"=w410:i64)  [unwired: 1 in, 1 out]
        n126 = call <vilib>:"Notify Event Complete.vi"("Completion Id"=w410, "Session in"=w411) -> ()  [unwired: 8 in, 2 out]
        n127 = To Variant(anything="Project Saved :- " ("string")) -> (Variant=w405:variant)
        n128 = call "Enqueue Message (Single).vi"("Message Data"=w405, "Message"="WriteConfig-InstrStudio", "Message Queue"=w408) -> ("error out"=w406:errorcluster, "dup Message Queue"=w407:refnum<queue>)  [unwired: 7 in]
      }
      event User Event {
        w412 = TRUE  # Priority Message? (F)
        # "Send acknowldement to InstrumentStudio"
        # "This event is triggered from InstrumentStudio when the project Stop All Outputs button is pressed"
        n129 = event-data() -> ("Completion Id"=w417:i64)  [unwired: 1 in]
        n130 = call <vilib>:"Notify Event Complete.vi"("Completion Id"=w417, "Session in"=w418) -> ()  [unwired: 8 in, 2 out]
        n131 = call "Enqueue Message (Single).vi"("Priority Message? (F)"=w412, "Message"="StopAllOutputs", "Message Queue"=w416) -> ("error out"=w413:errorcluster, "dup Message Queue"=w414:refnum<queue>)  [unwired: 7 in]
      }
      event User Event {
        w420 = bool[] [TRUE, TRUE]  # Priority Message? Array
        # "This event doesn't need acknowledgement from plugin"
        # "This event is triggered when softpanel/instrumentstudio is closed"
        n132 = event-data() -> ()  [unwired: 1 in, 1 out]
        n133 = call "Enqueue Message (Array).vi"("Priority Message? Array"=w420, "Message Array"=string[] ["Log Events", "Exit"], "Message Queue"=w421) -> ("error out"=w422:errorcluster, "dup Message Queue"=w423:refnum<queue>)  [unwired: 7 in]
      }
      event "height": Value Change {
        # "Captures value change in height and sends data to Message Handling Loop"
        n134 = event-data() -> ("NewVal"=w425:u32)  [unwired: 1 in]
        n135 = To Variant(anything=w425) -> (Variant=w424:variant)
        n136 = call "Enqueue Message (Single).vi"("Message Data"=w424, "Message"="Update Board Height", "Message Queue"=w427) -> ("error out"=w426:errorcluster, "dup Message Queue"=w428:refnum<queue>)  [unwired: 7 in]
      }
      event "width": Value Change {
        # "Captures value change in width and sends data to Message Handling Loop"
        n137 = event-data() -> ("NewVal"=w431:u32)  [unwired: 1 in]
        n138 = To Variant(anything=w431) -> (Variant=w430:variant)
        n139 = call "Enqueue Message (Single).vi"("Message Data"=w430, "Message"="Update Board Width", "Message Queue"=w433) -> ("error out"=w432:errorcluster, "dup Message Queue"=w434:refnum<queue>)  [unwired: 7 in]
      }
      event "update interval": Value Change {
        # "Captures value change in update interval and sends data to Message Handling Loop"
        n140 = event-data() -> ("NewVal"=w437:u32)  [unwired: 1 in]
        n141 = To Variant(anything=w437) -> (Variant=w436:variant)
        n142 = call "Enqueue Message (Single).vi"("Message Data"=w436, "Message"="Update Interval", "Message Queue"=w439) -> ("error out"=w438:errorcluster, "dup Message Queue"=w440:refnum<queue>)  [unwired: 7 in]
      }
      event "Log Events?": Value Change {
        # "Captures value change in Log Events and sends data to Message Handling Loop"
        n143 = event-data() -> ("NewVal"=w442:bool)  [unwired: 1 in]
        n144 = To Variant(anything=w442) -> (Variant=w445:variant)
        n145 = call "Enqueue Message (Single).vi"("Message Data"=w445, "Message"="Update Log Events", "Message Queue"=w444) -> ("dup Message Queue"=w443:refnum<queue>)  [unwired: 7 in, 1 out]
      }
      event "Start/Stop": Value Change {
        # "Captures value change in Start/Stop button and enqueues a state for Message Handling Loop"
        n146 = event-data() -> ("NewVal"=w448:bool)  [unwired: 1 in]
        n147 = To Variant(anything=w448) -> (Variant=w447:variant)
        n148 = call "Enqueue Message (Single).vi"("Message Data"=w447, "Message"="Update Start/Stop Game", "Message Queue"=w450) -> ("error out"=w449:errorcluster, "dup Message Queue"=w451:refnum<queue>)  [unwired: 7 in]
      }
      event Panel Close? {
        w453 = TRUE  # Priority Message? (F)
        # "Send the 'Confirm Quit' message if the user closes the panel of the VI. Discard the event so the 'Confirm Quit' message has a chance to run."
        n149 = event-data() -> ()  [unwired: 1 in, 1 out]
        n150 = call-poly "Enqueue Message.vi"("Priority Message? (F)"=w453, "Message"="Confirm Quit", "Message Queue"=w457) -> ("error out"=w456:errorcluster, "dup Message Queue"=w455:refnum<queue>)  [unwired: 7 in]
        n151 = event-data("Discard?"=TRUE) -> ()  [unwired: 1 in, 1 out]
      }
      event Application Instance Close {
        w463 = bool[] [TRUE, TRUE]  # Priority Message? Array
        # "Logs the events and exits the program."
        n152 = event-data() -> ()  [unwired: 1 in, 1 out]
        n153 = call "Enqueue Message (Array).vi"("Priority Message? Array"=w463, "Message Array"=string[] ["Log Events", "Exit"], "Message Queue"=w460) -> ("error out"=w459:errorcluster, "dup Message Queue"=w461:refnum<queue>)  [unwired: 7 in]
      }
      event User Event {
        w464 = TRUE  # Stop?
        # "The Message Handling Loop processed an \"Exit\" message, which fired this event to stop the Event Handling Loop."
        n154 = event-data() -> ()  [unwired: 1 in, 1 out]
      }
    }
    n155 = call "Error Handler - Event Handling Loop.vi"("error in (no error)"=w400, "Message Queue"=w398) -> ("dup error in"=w397:errorcluster)  [unwired: 8 in, 1 out]
  }
  n156 = Unregister For Events(event registration refnum=w18, error in=w17) -> (error out=w19:errorcluster)
  n157 = Merge Errors(w19, w23) -> (w20:errorcluster)
  n158 = call "Destroy User Event - Stop.vi"("error in (no error)"=w20, "User Event - Stop"=w16) -> ("error out"=w4:errorcluster)  [unwired: 9 in]
  n159 = call <vilib>:"Close Session.vi"("error in (no error)"=w4, "Session in"=w5) -> ("error out"=w3:errorcluster)  [unwired: 9 in]
  n160 = disable-structure shown="RUN_TIME_ENGINE==True" {
    disable-tunnel: w3 -> [_ _]
    frame condition #0 (active) {
    }
    frame condition #1 {
      # "Call Quit LabVIEW if running as a built application."
      n161 = Quit LabVIEW() -> ()  [unwired: 1 in]
    }
  }
